vi "TDMS Advanced Asynchronous Read Speed Test.vi"() -> ()   [LabVIEW 2023]
doc: "This example demonstrates how to benchmark the streaming performance when you use the TDMS Advanced Asynchronous I/O functions to read data from a .tdms file. This VI measures the time it takes to continuously read data from a file and calculates the average data throughput in bytes/second."
panel:
  out "Total Number of Reads":u64
  in  "Read Block Size (bytes)":u64=4194304 step=1048576
  in  "Number of Buffers (4)":u32=4 step=1048576
  in  "Disable Buffering? (T)":bool=TRUE
  out "Bytes/second":dbl format="%#_4p"
  out "Current Number of Reads":i32
  # "Overview: Demonstrates how to benchmark the streaming performance when you use the TDMS Advanced Asynchronous Read  function to read data from a .tdms file.\nInstructions:\n1. Make sure you have already run TDMS Advanced Asynchronous Write Speed Test.vi.\n2. Run the VI.\n3. Delete the TDMS file (located at [LabVIEW Data]\\Example TDMS Asynchronous Speed Test Data.tdms) when you are done."
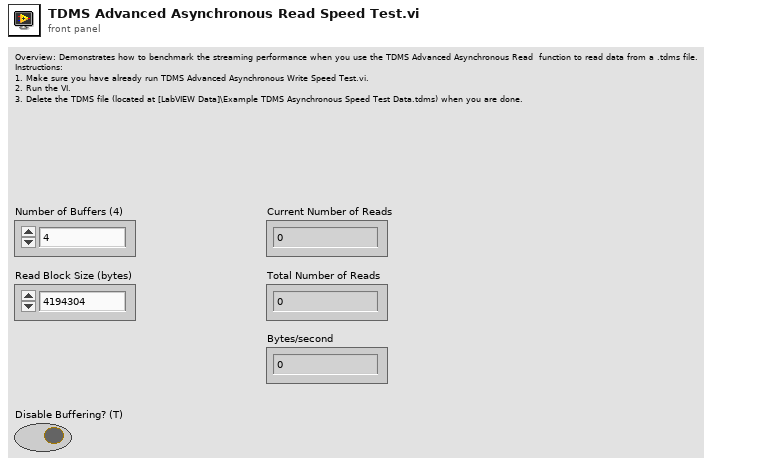
[diagram p1: front panel]
types:
  T1 = enum16{"open", "open or create", "create or replace", "create", "open (read-only)"}
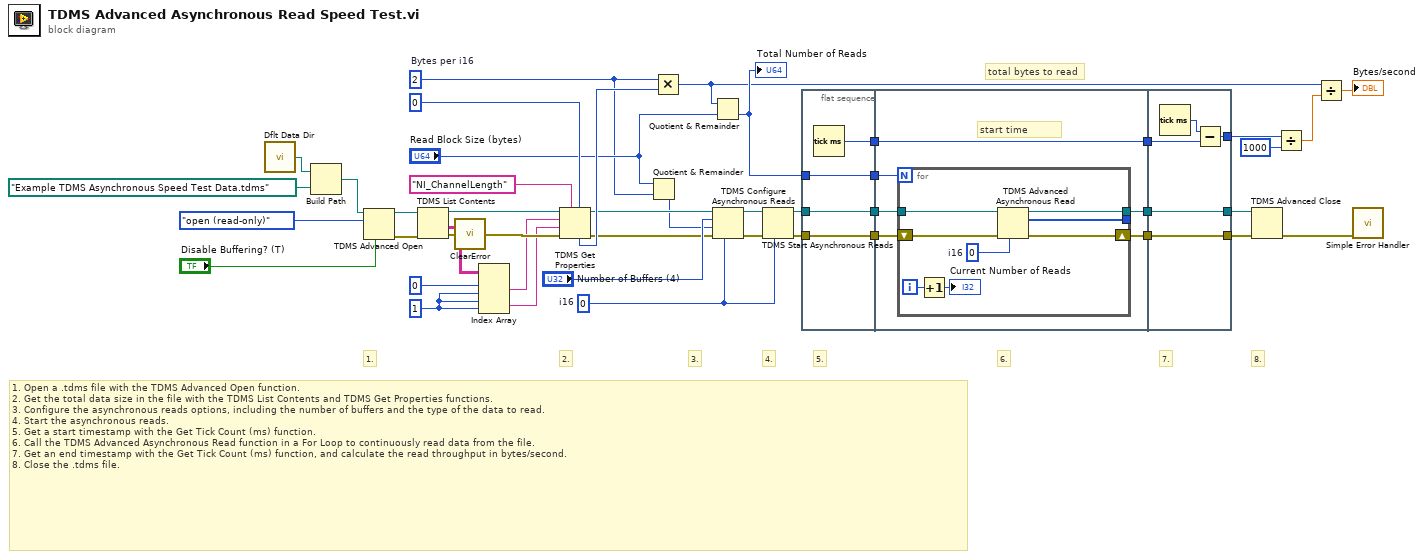
[diagram p0: block diagram]
diagram:
  w26 = 1 ("disabled index (col)")
  w10 = u64 2  # Bytes per i16
  w29 = i16 0  # i16
  # "total bytes to read"
  # "8."
  # "7."
  # "3."
  # "6."
  # "5."
  # "4."
  # "2."
  # "1."
  # "1. Open a .tdms file with the TDMS Advanced Open function.\n2. Get the total data size in the file with the TDMS List Contents and TDMS Get Properties functions. \n3. Configure the asynchronous reads options, including the number of buffers and the type of the data to read.\n4. Start the asynchronous reads.\n5. Get a start timestamp with the Get Tick Count (ms) function.\n6. Call the TDMS Advanced Asynchronous Read function in a For Loop to continuously read data from the file.\n7. Get an end timestamp with the Get Tick Count (ms) function, and calculate the read throughput in bytes/second.\n8. Close the .tdms file."
  n1 = call <vilib>:"Dflt Data Dir.vi"() -> ("App:Default Data Directory"=w3:path)
  n2 = Build Path(base path=w3, name or relative path=path "Example TDMS Asynchronous Speed Test Data.tdms") -> (appended path=w2:path)
  n3 = TDMS Advanced Open(6:"Disable Buffering? (T)", 10:T1."open (read-only)" ("Operation"), 11:w2) -> (0:w18:errorcluster, 3:w17:refnum<k34>)  [unwired: 2 in, 1 out]
  n4 = TDMS List Contents(4:w18, 7:w17) -> (0:w1:errorcluster, 1:w28:string[][], 3:w24:refnum<k34>)  [unwired: 1 in, 1 out]
  n5 = call <vilib>:"ClearError.vi"("error in (no error)"=w1) -> ("error out"=w25:errorcluster)
  n6 = Index Array(array=w28, index (row) #1=0 ("index (row)"), index (col) #1=w26, index (row) #2=w26, index (col) #2=w26) -> (element #1=w23:string, element #2=w22:string)
  n7 = TDMS Get Properties(5:0, 7:"NI_ChannelLength" ("property name"), 8:w25, 9:w22, 10:w23, 11:w24) -> (0:w15:errorcluster, 3:w16:refnum<k34>, 4:w19:i32)  [unwired: 3 out]
  n8 = Quotient & Remainder(x="Read Block Size (bytes)", y=w10) -> (floor(x/y)=w11:u64)  [unwired: 1 out]
  n9 = Multiply(x=w10, y=w19) -> (x*y=w6:u64)
  n10 = Quotient & Remainder(x=w6, y="Read Block Size (bytes)") -> (floor(x/y)=w13:u64)  [unwired: 1 out]
  "Total Number of Reads" <- w13
  n11 = TDMS Configure Asynchronous Reads(6:w29, 8:w15, 9:w11, 10:"Number of Buffers (4)", 11:w16) -> (0:w34:errorcluster, 3:w33:refnum<k34>)  [unwired: 1 in]
  n12 = TDMS Start Asynchronous Reads(6:w29, 8:w34, 11:w33) -> (0:w31:errorcluster, 3:w32:refnum<k34>)  [unwired: 1 in]
  n13 = flat-sequence {
    tunnel: w31 -> [w49]
    tunnel: [w49] -> w45
    tunnel: w32 -> [w48]
    tunnel: [w48] -> w44
    tunnel: [w47] -> w43
    tunnel: [w46] -> w14
    tunnel: w13 -> [w46]
    tunnel: w45 -> [w55]
    tunnel: w44 -> [w54]
    tunnel: w43 -> [w53]
    tunnel: [w53] -> w42
    tunnel: [w52] -> w41
    tunnel: [w51] -> w40
    tunnel: w14 -> [w50]
    tunnel: w42 -> [w67]
    tunnel: w41 -> [w66]
    tunnel: [w66] -> w38
    tunnel: [w65] -> w37
    tunnel: w40 -> [w65]
    tunnel: [w64] -> w8
    frame #0 {
      n14 = Tick Count (ms)() -> (millisecond timer value=w47:u32)
    }
    frame #1 {
      # "start time"
      n15 = for {
        N: w50 -> [_]
        tunnel: [w59] -> w52
        shift-right: [w63] -> w51
        shift-left: w55 -> [w62]
        tunnel: w54 -> [w56]
        tunnel: [w58] -> _
        i -> [w61]
        w57 = i16 0  # i16
        n16 = Increment(x=w61) -> (x+1=→"Current Number of Reads":i32)
        n17 = TDMS Advanced Asynchronous Read(6:w57, 8:w62, 11:w56) -> (0:w63:errorcluster, 2:w58:i16[], 3:w59:refnum<k34>)  [unwired: 1 out]
      }
    }
    frame #2 {
      n18 = Tick Count (ms)() -> (millisecond timer value=w68:u32)
      n19 = Subtract(x=w68, y=w67) -> (x-y=w64:u32)
    }
  }
  n20 = TDMS Advanced Close(8:w37, 11:w38) -> (0:w39:errorcluster)  [unwired: 2 in, 1 out]
  n21 = Divide(x=w8, y=u32 1000) -> (x/y=w5:dbl)
  n22 = Divide(x=w6, y=w5) -> (x/y=→"Bytes/second":dbl)
  n23 = call <vilib>:"Simple Error Handler.vi"("error in (no error)"=w39) -> ()  [unwired: 1 in, 8 out]
